vi "SimulatedScope SimulatedFGen Test.vi"(8 "Error In":errorcluster) -> (0 "Error Out":errorcluster)   [LabVIEW 2023]
uses:
  Measure and Stimulus Subsystems/Measure and Stimulus Subsystems.lvclass
panel:
  in  "Stop":bool
  out "Photosensor Waveform Chart":waveform(dbl)(graph)
  out "Powersensor Scalar":dbl
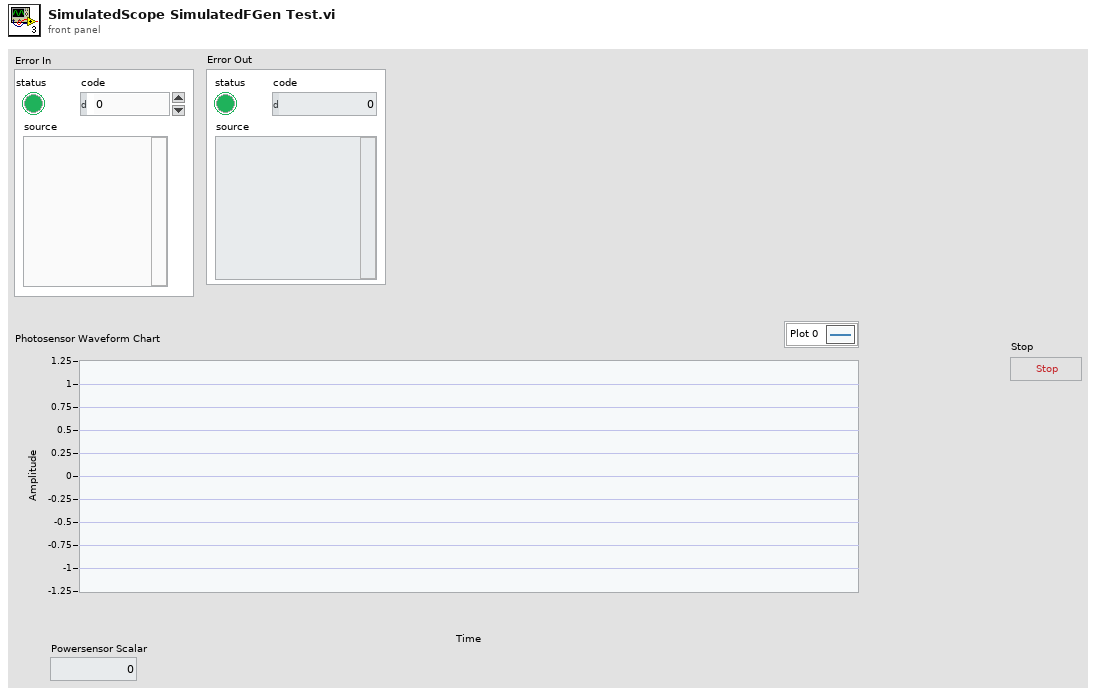
[diagram p1: front panel]
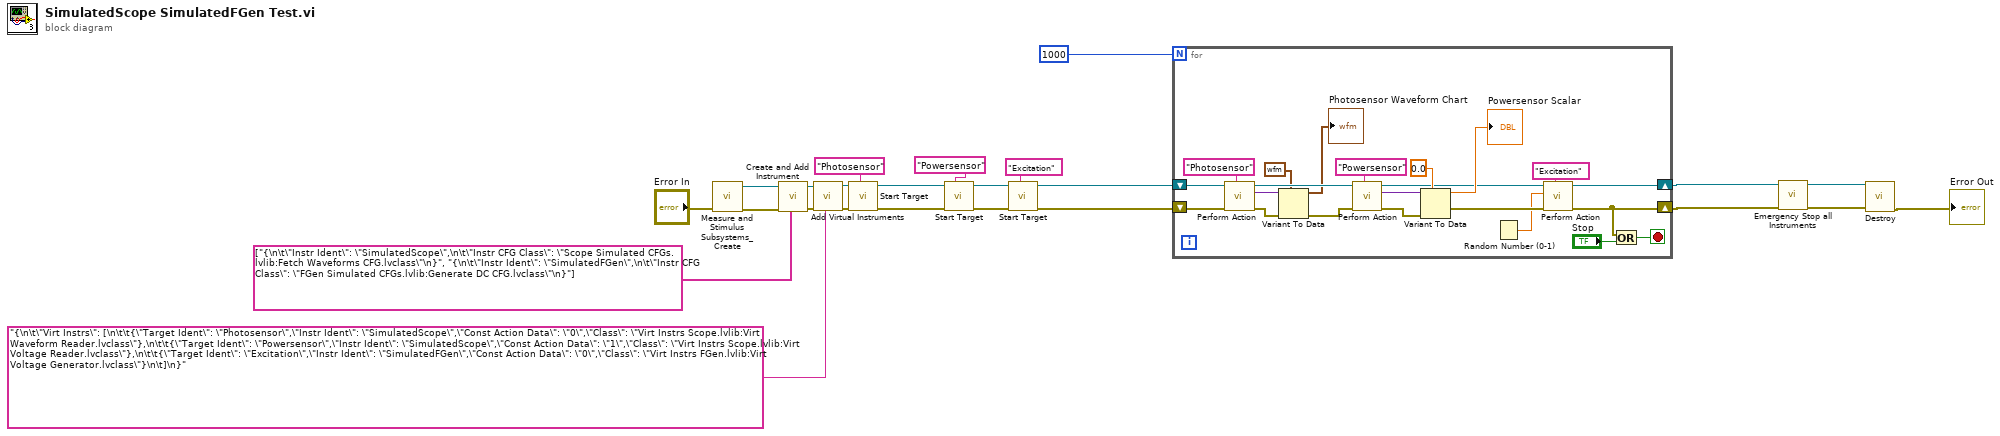
[diagram p0: block diagram]
diagram:
  n1 = call "Measure and Stimulus Subsystems_Create.vi"("Error In"="Error In") -> ("Error Out"=w23:errorcluster, "reference out"=w24:refnum<class "Measure and Stimulus Subsystems.lvclass">)  [unwired: 9 in]
  n2 = call "Create and Add Instrument.vi"("Physical Intr Configs"=string[] ["{\n\t\"Instr Ident\": \"SimulatedScope\",\n\t\"Instr CFG Class\": \"Scope Simulated CFGs.lvlib:Fetch Waveforms CFG.lvclass\"\n}", "{\n\t\"Instr Ident\": \"SimulatedFGen\",\n\t\"Instr CFG Class\": \"FGen Simulated CFGs.lvlib:Generate DC CFG.lvclass\"\n}"], "Error In"=w23, "reference in"=w24) -> ("Error Out"=w22:errorcluster, "reference out"=w3:refnum<class "Measure and Stimulus Subsystems.lvclass">)  [unwired: 7 in]
  n3 = call "Add Virtual Instruments.vi"("<JSON CFG>"="{\n\t\"Virt Instrs\": [\n\t\t{\"Target Ident\": \"Photosensor\",\"Instr Ident\": \"SimulatedScope\",\"Const Action Data\": \"0\",\"Class\": \"Virt Instrs Scope.lvlib:Virt Waveform Reader.lvclass\"},\n\t\t{\"Target Ident\": \"Powersensor\",\"Instr Ident\": \"SimulatedScope\",\"Const Action Data\": \"1\",\"Class\": \"Virt Instrs Scope.lvlib:Virt Voltage Reader.lvclass\"},\n\t\t{\"Target Ident\": \"Excitation\",\"Instr Ident\": \"SimulatedFGen\",\"Const Action Data\": \"0\",\"Class\": \"Virt Instrs FGen.lvlib:Virt Voltage Generator.lvclass\"}\n\t]\n}", "Error In"=w22, "reference in"=w3) -> ("Error Out"=w4:errorcluster, "reference out"=w2:refnum<class "Measure and Stimulus Subsystems.lvclass">)  [unwired: 7 in]
  n4 = call "Start Target.vi"("Target Ident"="Photosensor" ("Target Identifier"), "Error In"=w4, "reference in"=w2) -> ("Error Out"=w13:errorcluster, "reference out"=w10:refnum<class "Measure and Stimulus Subsystems.lvclass">)  [unwired: 7 in]
  n5 = call "Start Target.vi"("Target Ident"="Powersensor" ("Target Identifier"), "Error In"=w13, "reference in"=w10) -> ("Error Out"=w11:errorcluster, "reference out"=w9:refnum<class "Measure and Stimulus Subsystems.lvclass">)  [unwired: 7 in]
  n6 = call "Start Target.vi"("Target Ident"="Excitation", "Error In"=w11, "reference in"=w9) -> ("Error Out"=w21:errorcluster, "reference out"=w6:refnum<class "Measure and Stimulus Subsystems.lvclass">)  [unwired: 7 in]
  n7 = for {
    N: 1000 -> [_]
    shift-right: [w29] -> w16
    shift-left: w21 -> [w41]
    shift-right: [w27] -> w19
    shift-left: w6 -> [w40]
    stop <- w30 stop-if-true
    n8 = call "Perform Action.vi"("Target Ident"="Photosensor" ("Target Identifier"), "Error In"=w41, "reference in"=w40) -> ("Error Out"=w44:errorcluster, "Output"=w38:variant, "reference out"=w45:refnum<class "Measure and Stimulus Subsystems.lvclass">)  [unwired: 6 in]
    n9 = Variant To Data(error in=w44, type=waveform(dbl) {"t0"=timestamp(0 s since 1904-01-01), "dt"=1.0, "Y"=[]} ("Waveform"), Variant=w38) -> (data=→"Photosensor Waveform Chart":waveform(dbl), error out=w39:errorcluster)
    n10 = call "Perform Action.vi"("Target Ident"="Powersensor" ("Target Identifier"), "Error In"=w39, "reference in"=w45) -> ("Error Out"=w42:errorcluster, "Output"=w36:variant, "reference out"=w28:refnum<class "Measure and Stimulus Subsystems.lvclass">)  [unwired: 6 in]
    n11 = Variant To Data(error in=w42, type=0.0, Variant=w36) -> (data=→"Powersensor Scalar":dbl, error out=w31:errorcluster)
    n12 = Random Number (0-1)() -> (number: 0 to 1=w25:dbl)
    n13 = call "Perform Action.vi"("Target Ident"="Excitation", "Error In"=w31, "Input"=w25, "reference in"=w28) -> ("Error Out"=w29:errorcluster, "reference out"=w27:refnum<class "Measure and Stimulus Subsystems.lvclass">)  [unwired: 5 in, 1 out]
    n14 = Or(x=w29, y="Stop") -> (x .or. y?=w30:bool)
  }
  n15 = call "Emergency Stop all Instruments.vi"("Error In"=w16, "reference in"=w19) -> ("Error Out"=w20:errorcluster, "reference out"=w18:refnum<class "Measure and Stimulus Subsystems.lvclass">)  [unwired: 8 in]
  n16 = call "Destroy.vi"("Error In"=w20, "reference in"=w18) -> ("Error Out"=→"Error Out":errorcluster)  [unwired: 8 in, 1 out]
